vi "Apply Signal Transition.vi"(0 "signal configuration and state in":refnum<class "SV Signal.lvclass">, 5 "waveform":waveform(dbl)={"t0"=timestamp(0 s since 1904-01-01), "dt"=0.001, "Y"=[]}, 11 "error in (no error)":errorcluster) -> (4 "signal configuration and state out":refnum<class "SV Signal.lvclass">, 6 "profiled waveform":waveform(dbl)={"t0"=timestamp(0 s since 1904-01-01), "dt"=0.001, "Y"=[]}, 15 "error out":errorcluster)   [LabVIEW 2017, in "SV Signal.lvclass"]
uses:
  <vilib>/addons/_NISVFA/_Generation/Signal Generation/SV Signal/SV Signal.lvclass
  <vilib>/addons/_NISVFA/_Generation/Signal Generation/SV Signal/SV Signal.lvclass/SV Signal.ctl
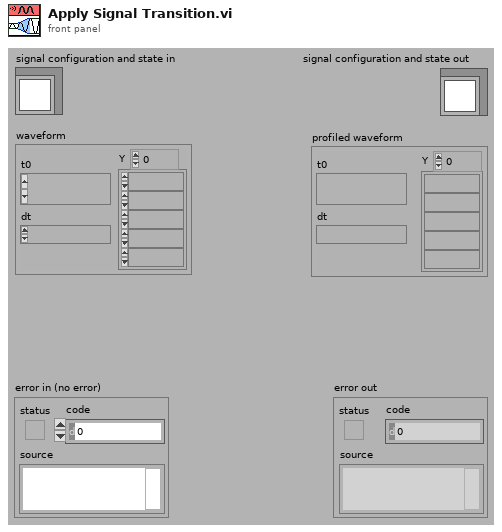
[diagram p1: front panel]
types:
  T1 = typedef "SV Signal.lvclass/sv_System Timing Model.ctl" = i64
  T2 = typedef "SV Signal.lvclass/sv_Generation State.ctl" = enum16{"Idle", "Ramp Up", "Pre-Measurement Settling", "Measurement", "Post-Measurement Settling", "Discrete Sweep Transition", "Ramp Down", "Update"}
  T3 = cluster{"system timing model":T1, "state":cluster{"RESET":bool, "generator timestamp":timestamp, "elapsed seconds":dbl, "elapsed samples":u64, "generation state":T2, "time offset at state":dbl, "samples generated at state":u64, "signal state":variant}, "duration of state":dbl, "samples remaining at state":i32}
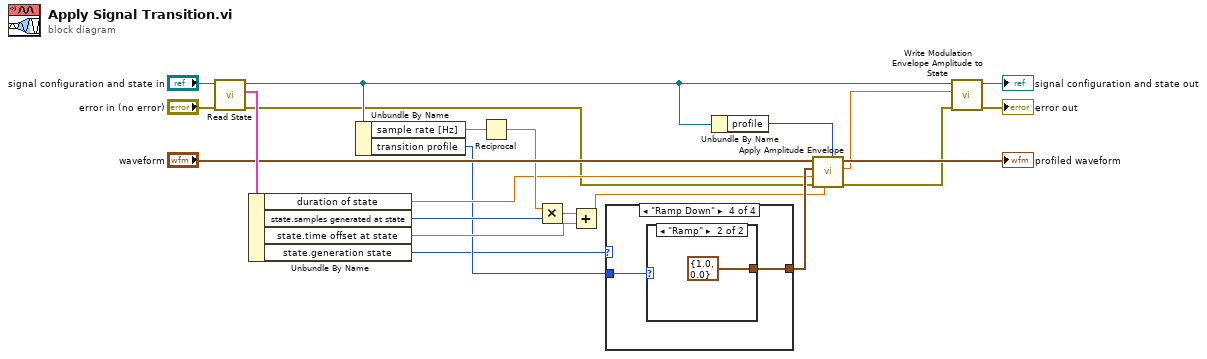
[diagram p0: block diagram]
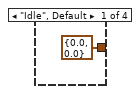
[diagram p2: hidden frame]
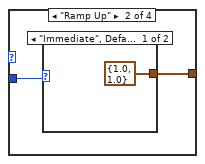
[diagram p3: hidden frame]
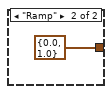
[diagram p4: hidden frame]
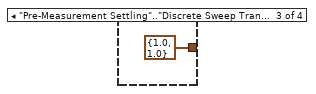
[diagram p5: hidden frame]
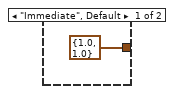
[diagram p6: hidden frame]
diagram:
  n1 = call <vilib>:"Read State.vi"("error in (no error)"="error in (no error)", "signal configuration"="signal configuration and state in") -> ("error out"=w3:errorcluster, "generator state"=w19:T3, "signal configuration"=w4:refnum<class "SV Signal.lvclass">)  [unwired: 7 in]
  n2 = Unbundle By Name(w19) -> ("duration of state"=w6:dbl, "state.samples generated at state"=w8:u64, "state.time offset at state"=w7:dbl, "state.generation state"=w1:T2)
  n3 = Unbundle By Name(w4) -> ("sample rate [Hz]"=w5:dbl, "transition profile"=w2:enum16{"Immediate", "Next optimum", "Ramp"})
  n4 = Reciprocal(x=w5) -> (1/x=w12:dbl)
  n5 = Multiply(x=w12, y=w8) -> (x*y=w22:dbl)
  n6 = Add(x=w22, y=w7) -> (x+y=w13:dbl)
  n7 = case shown="\"Ramp Down\"" w1 {
    tunnel: [cluster{"start":dbl, "stop":dbl} {"start"=0.0, "stop"=0.0} ("endpoints") w25 cluster{"start":dbl, "stop":dbl} {"start"=1.0, "stop"=1.0} ("endpoints") w30] -> w14
    tunnel: w2 -> [_ w24 _ w29]
    frame "Idle", Default {
    }
    frame "Ramp Up" {
      n8 = case shown="\"Immediate\", Default" w24 {
        tunnel: [cluster{"start":dbl, "stop":dbl} {"start"=1.0, "stop"=1.0} ("endpoints") cluster{"start":dbl, "stop":dbl} {"start"=0.0, "stop"=1.0} ("endpoints")] -> w25
        frame "Immediate", Default {
        }
        frame "Ramp" {
        }
      }
    }
    frame "Pre-Measurement Settling".."Discrete Sweep Transition" {
    }
    frame "Ramp Down" {
      n9 = case shown="\"Ramp\"" w29 {
        tunnel: [cluster{"start":dbl, "stop":dbl} {"start"=1.0, "stop"=1.0} ("endpoints") cluster{"start":dbl, "stop":dbl} {"start"=1.0, "stop"=0.0} ("endpoints")] -> w30
        frame "Immediate", Default {
        }
        frame "Ramp" {
        }
      }
    }
  }
  n10 = Unbundle By Name(w4) -> ("profile"=w16:enum16{"Linear", "Half cosine"})
  n11 = call <vilib>:"Apply Amplitude Envelope.vi"("profile"=w16, "time elapsed at transition"=w13, "error in (no error)"=w3, "duration"=w6, "amplitude modulation"=w14, "waveform in"="waveform") -> ("error out"=w9:errorcluster, "amplitude envelope last value"=w17:dbl, "waveform out"=→"profiled waveform":waveform(dbl))  [unwired: 3 in]
  n12 = call <vilib>:"Write Modulation Envelope Amplitude to State.vi"("error in (no error)"=w9, "modulation envelope amplitude"=w17, "SV Signal in"=w4) -> ("error out"=→"error out":errorcluster, "SV Signal out"=→"signal configuration and state out":refnum<class "SV Signal.lvclass">)  [unwired: 7 in]
